vi "Read Limelight Values.vi"   [LabVIEW 2019]
uses:
  <vilib>/Rock Robotics/Network Tables/NT Read Number.vi
  Framework/Robot Global Data.vi
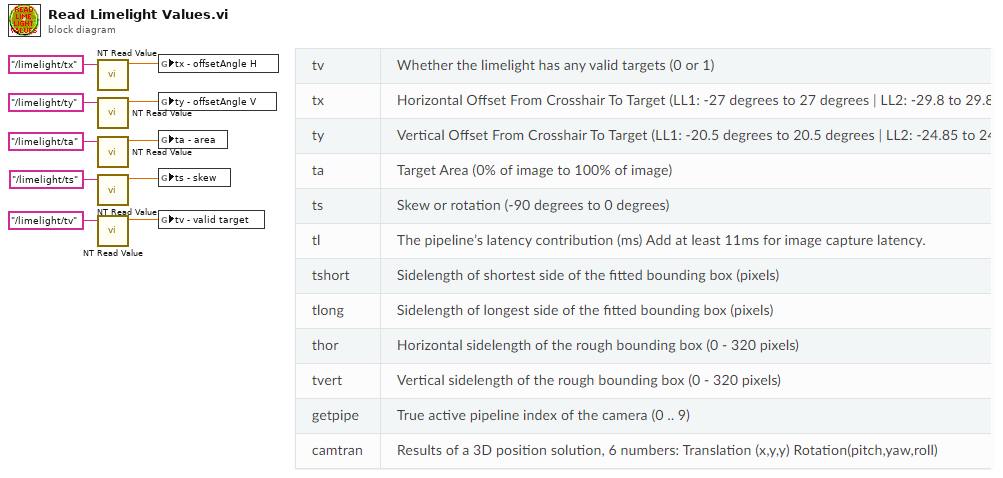
[diagram p0: block diagram]
diagram:
  n1 = call-poly <vilib>:"NT Read Value.vi"("Name"="/limelight/tx") -> ("Numeric"=w6:dbl)  [unwired: 9 in, 1 out]
  n2 = call-poly <vilib>:"NT Read Value.vi"("Name"="/limelight/ty") -> ("Numeric"=w4:dbl)  [unwired: 9 in, 1 out]
  n3 = call-poly <vilib>:"NT Read Value.vi"("Name"="/limelight/ta") -> ("Numeric"=w3:dbl)  [unwired: 9 in, 1 out]
  n4 = call-poly <vilib>:"NT Read Value.vi"("Name"="/limelight/ts") -> ("Numeric"=w5:dbl)  [unwired: 9 in, 1 out]
  n5 = call-poly <vilib>:"NT Read Value.vi"("Name"="/limelight/tv") -> ("Numeric"=w2:dbl)  [unwired: 9 in, 1 out]
  n6 = global write "Robot Global Data.vi" "tx - offsetAngle H"(w6) -> ()
  n7 = global write "Robot Global Data.vi" "ty - offsetAngle V"(w4) -> ()
  n8 = global write "Robot Global Data.vi" "ta - area"(w3) -> ()
  n9 = global write "Robot Global Data.vi" "ts - skew"(w5) -> ()
  n10 = global write "Robot Global Data.vi" "tv - valid target"(w2) -> ()
